vi "VI Tree.vi"   [LabVIEW 2014, in "Agilent NA.lvlib"]
doc: "The VI Tree displays all the user-callable VIs of the instrument driver in an organized table."
uses:
  Agilent NA.lvlib
panel:
  # "NA"
  # "1.0.1"
  # "SEE DIAGRAM\nFOR VI Tree"
  # "© 2014 Agilent Technologies, Inc."
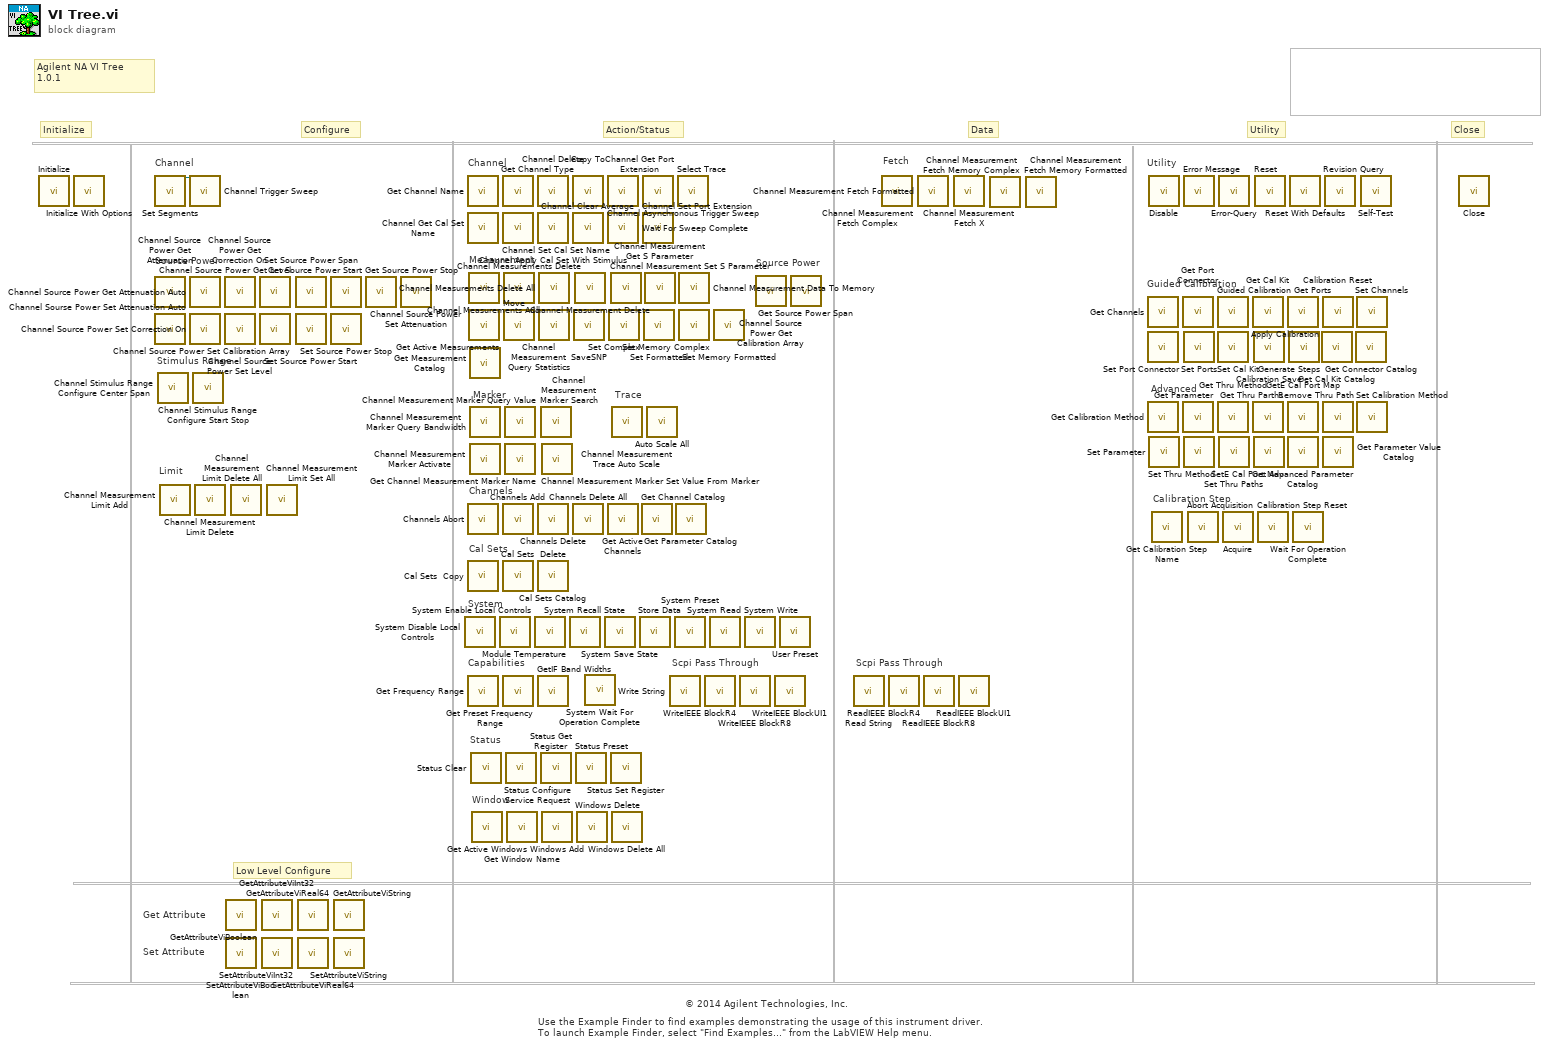
[diagram p0: block diagram]
diagram:
  # "Marker"
  # "Cal Sets"
  # "Utility"
  # "Fetch"
  # "Scpi Pass Through"
  # "Source Power"
  # "Channel"
  # "Status"
  # "Set Attribute"
  # "Get Attribute"
  # "Low Level Configure"
  # "Action/Status"
  # "Agilent NA VI Tree\n1.0.1"
  # "© 2014 Agilent Technologies, Inc."
  # "Close"
  # "Data"
  # "Configure"
  # "Initialize"
  # "Use the Example Finder to find examples demonstrating the usage of this instrument driver.\nTo launch Example Finder, select \"Find Examples...\" from the LabVIEW Help menu."
  # "Window"
  # "Utility"
  # "Scpi Pass Through"
  # "Capabilities"
  # "System"
  # "Calibration Step"
  # "Advanced"
  # "Guided Calibration"
  # "Channels"
  # "Stimulus Range"
  # "Source Power"
  # "Trace"
  # "Limit"
  # "Measurement"
  # "Channel"
  n1 = call "Initialize.vi"() -> ()  [unwired: 10 in, 2 out]
  n2 = call "Initialize With Options.vi"() -> ()  [unwired: 10 in, 2 out]
  n3 = call "Set Segments.vi"() -> ("instrument handle out"=w1:refnum<k15>)  [unwired: 26 in, 1 out]
  n4 = call "Channel Source Power Get Attenuation.vi"() -> ()  [unwired: 9 in, 3 out]
  n5 = call "Channel Sourse Power Set Attenuation Auto.vi"() -> ()  [unwired: 10 in, 2 out]
  n6 = call "Channel Stimulus Range Configure Center Span.vi"() -> ()  [unwired: 10 in, 2 out]
  n7 = call "Channel Measurement Limit Add.vi"() -> ()  [unwired: 10 in, 2 out]
  n8 = call "Channel Trigger Sweep.vi"("instrument handle"=w1) -> ()  [unwired: 9 in, 2 out]
  n9 = call "Channel Source Power Get Attenuation Auto.vi"() -> ()  [unwired: 9 in, 3 out]
  n10 = call "Channel Source Power Set Correction On.vi"() -> ()  [unwired: 10 in, 2 out]
  n11 = call "Channel Stimulus Range Configure Start Stop.vi"() -> ()  [unwired: 10 in, 2 out]
  n12 = call "Channel Measurement Limit Delete.vi"() -> ()  [unwired: 10 in, 2 out]
  n13 = call "Channel Source Power Get Correction On.vi"() -> ()  [unwired: 9 in, 3 out]
  n14 = call "Channel Source Power Set Level.vi"() -> ()  [unwired: 10 in, 2 out]
  n15 = call "GetAttributeViBoolean.vi"() -> ()  [unwired: 9 in, 3 out]
  n16 = call "SetAttributeViBoolean.vi"() -> ()  [unwired: 10 in, 2 out]
  n17 = call "Channel Measurement Limit Delete All.vi"() -> ()  [unwired: 10 in, 2 out]
  n18 = call "Channel Source Power Get Level.vi"() -> ()  [unwired: 9 in, 3 out]
  n19 = call "Channel Source Power Set Calibration Array.vi"() -> ()  [unwired: 9 in, 3 out]
  n20 = call "GetAttributeViInt32.vi"() -> ()  [unwired: 9 in, 3 out]
  n21 = call "SetAttributeViInt32.vi"() -> ()  [unwired: 10 in, 2 out]
  n22 = call "Channel Measurement Limit Set All.vi"() -> ()  [unwired: 26 in, 2 out]
  n23 = call "Set Source Power Span.vi"() -> ()  [unwired: 10 in, 2 out]
  n24 = call "Set Source Power Start.vi"() -> ()  [unwired: 10 in, 2 out]
  n25 = call "GetAttributeViReal64.vi"() -> ()  [unwired: 9 in, 3 out]
  n26 = call "SetAttributeViReal64.vi"() -> ()  [unwired: 10 in, 2 out]
  n27 = call "Get Source Power Start.vi"() -> ()  [unwired: 9 in, 3 out]
  n28 = call "Set Source Power Stop.vi"() -> ()  [unwired: 10 in, 2 out]
  n29 = call "GetAttributeViString.vi"() -> ()  [unwired: 9 in, 3 out]
  n30 = call "SetAttributeViString.vi"() -> ()  [unwired: 10 in, 2 out]
  n31 = call "Get Source Power Stop.vi"() -> ()  [unwired: 9 in, 3 out]
  n32 = call "Channel Source Power Set Attenuation.vi"() -> ()  [unwired: 10 in, 2 out]
  n33 = call "System Disable Local Controls.vi"() -> ()  [unwired: 10 in, 2 out]
  n34 = call "Get Channel Name.vi"() -> ()  [unwired: 9 in, 3 out]
  n35 = call "Channel Get Cal Set Name.vi"() -> ()  [unwired: 9 in, 3 out]
  n36 = call "Channels Abort.vi"() -> ()  [unwired: 10 in, 2 out]
  n37 = call "Cal Sets  Copy.vi"() -> ()  [unwired: 10 in, 2 out]
  n38 = call "Get Frequency Range.vi"() -> ()  [unwired: 8 in, 4 out]
  n39 = call "Channel Measurements Add.vi"() -> ()  [unwired: 9 in, 3 out]
  n40 = call "Get Active Measurements.vi"() -> ()  [unwired: 8 in, 4 out]
  n41 = call "Get Measurement Catalog.vi"() -> ()  [unwired: 9 in, 3 out]
  n42 = call "Channel Measurement Marker Query Bandwidth.vi"() -> ()  [unwired: 6 in, 6 out]
  n43 = call "Channel Measurement Marker Activate.vi"() -> ()  [unwired: 10 in, 2 out]
  n44 = call "Status Clear.vi"() -> ()  [unwired: 10 in, 2 out]
  n45 = call "Get Active Windows.vi"() -> ()  [unwired: 8 in, 4 out]
  n46 = call "System Enable Local Controls.vi"() -> ()  [unwired: 10 in, 2 out]
  n47 = call "Get Channel Type.vi"() -> ()  [unwired: 9 in, 3 out]
  n48 = call "Channel Set Cal Set Name.vi"() -> ()  [unwired: 10 in, 2 out]
  n49 = call "Channels Add.vi"() -> ()  [unwired: 9 in, 3 out]
  n50 = call "Cal Sets  Delete.vi"() -> ()  [unwired: 10 in, 2 out]
  n51 = call "Get Preset Frequency Range.vi"() -> ()  [unwired: 8 in, 4 out]
  n52 = call "Channel Measurements Delete.vi"() -> ()  [unwired: 10 in, 2 out]
  n53 = call "Move.vi"() -> ()  [unwired: 10 in, 2 out]
  n54 = call "Channel Measurement Marker Query Value.vi"() -> ()  [unwired: 8 in, 4 out]
  n55 = call "Get Channel Measurement Marker Name.vi"() -> ()  [unwired: 9 in, 3 out]
  n56 = call "Status Configure Service Request.vi"() -> ()  [unwired: 10 in, 2 out]
  n57 = call "Get Window Name.vi"() -> ()  [unwired: 9 in, 3 out]
  n58 = call "Module Temperature.vi"() -> ()  [unwired: 9 in, 3 out]
  n59 = call "Channel Delete.vi"() -> ()  [unwired: 10 in, 2 out]
  n60 = call "Channel Apply Cal Set With Stimulus.vi"() -> ()  [unwired: 10 in, 2 out]
  n61 = call "Channels Delete.vi"() -> ()  [unwired: 10 in, 2 out]
  n62 = call "Cal Sets Catalog.vi"() -> ()  [unwired: 9 in, 3 out]
  n63 = call "GetIF Band Widths.vi"() -> ()  [unwired: 8 in, 4 out]
  n64 = call "Channel Measurements Delete All.vi"() -> ()  [unwired: 10 in, 2 out]
  n65 = call "Channel Measurement Query Statistics.vi"() -> ()  [unwired: 9 in, 3 out]
  n66 = call "Channel Measurement Marker Search.vi"() -> ()  [unwired: 10 in, 2 out]
  n67 = call "Status Get Register.vi"() -> ()  [unwired: 9 in, 3 out]
  n68 = call "Channel Measurement Marker Set Value From Marker.vi"() -> ()  [unwired: 10 in, 2 out]
  n69 = call "Windows Add.vi"() -> ()  [unwired: 10 in, 2 out]
  n70 = call "System Recall State.vi"() -> ()  [unwired: 10 in, 2 out]
  n71 = call "Copy To.vi"() -> ()  [unwired: 10 in, 2 out]
  n72 = call "Channel Clear Average.vi"() -> ()  [unwired: 10 in, 2 out]
  n73 = call "Channels Delete All.vi"() -> ()  [unwired: 10 in, 2 out]
  n74 = call "SaveSNP.vi"() -> ()  [unwired: 10 in, 2 out]
  n75 = call "Channel Measurement Delete.vi"() -> ()  [unwired: 10 in, 2 out]
  n76 = call "Status Preset.vi"() -> ()  [unwired: 10 in, 2 out]
  n77 = call "Windows Delete.vi"() -> ()  [unwired: 10 in, 2 out]
  n78 = call "System Wait For Operation Complete.vi"() -> ()  [unwired: 10 in, 2 out]
  n79 = call "System Save State.vi"() -> ()  [unwired: 10 in, 2 out]
  n80 = call "Channel Asynchronous Trigger Sweep.vi"() -> ()  [unwired: 10 in, 2 out]
  n81 = call "Wait For Sweep Complete.vi"() -> ()  [unwired: 10 in, 2 out]
  n82 = call "Get Active Channels.vi"() -> ()  [unwired: 8 in, 4 out]
  n83 = call "Set Complex.vi"() -> ()  [unwired: 10 in, 2 out]
  n84 = call "Channel Measurement Set S Parameter.vi"() -> ()  [unwired: 10 in, 2 out]
  n85 = call "Status Set Register.vi"() -> ()  [unwired: 10 in, 2 out]
  n86 = call "Channel Measurement Trace Auto Scale.vi"() -> ()  [unwired: 10 in, 2 out]
  n87 = call "Windows Delete All.vi"() -> ()  [unwired: 10 in, 2 out]
  n88 = call "Store Data.vi"() -> ()  [unwired: 10 in, 2 out]
  n89 = call "Get Channel Catalog.vi"() -> ()  [unwired: 9 in, 3 out]
  n90 = call "Channel Get Port Extension.vi"() -> ()  [unwired: 9 in, 3 out]
  n91 = call "Channel Set Port Extension.vi"() -> ()  [unwired: 10 in, 2 out]
  n92 = call "Set Formatted.vi"() -> ()  [unwired: 10 in, 2 out]
  n93 = call "Channel Measurement Get S Parameter.vi"() -> ()  [unwired: 8 in, 4 out]
  n94 = call "Auto Scale All.vi"() -> ()  [unwired: 10 in, 2 out]
  n95 = call "Write String.vi"() -> ()  [unwired: 10 in, 2 out]
  n96 = call "System Preset.vi"() -> ()  [unwired: 10 in, 2 out]
  n97 = call "Get Parameter Catalog.vi"() -> ()  [unwired: 9 in, 3 out]
  n98 = call "Select Trace.vi"() -> ()  [unwired: 10 in, 2 out]
  n99 = call "Channel Measurement Data To Memory.vi"() -> ()  [unwired: 10 in, 2 out]
  n100 = call "Set Memory Complex.vi"() -> ()  [unwired: 10 in, 2 out]
  n101 = call "WriteIEEE BlockR4.vi"() -> ()  [unwired: 10 in, 2 out]
  n102 = call "System Read.vi"() -> ()  [unwired: 8 in, 4 out]
  n103 = call "Set Memory Formatted.vi"() -> ()  [unwired: 10 in, 2 out]
  n104 = call "WriteIEEE BlockR8.vi"() -> ()  [unwired: 10 in, 2 out]
  n105 = call "System Write.vi"() -> ()  [unwired: 10 in, 2 out]
  n106 = call "Channel Source Power Get Calibration Array.vi"() -> ()  [unwired: 8 in, 4 out]
  n107 = call "WriteIEEE BlockUI1.vi"() -> ()  [unwired: 10 in, 2 out]
  n108 = call "User Preset.vi"() -> ()  [unwired: 10 in, 2 out]
  n109 = call "Get Source Power Span.vi"() -> ()  [unwired: 9 in, 3 out]
  n110 = call "Read String.vi"() -> ()  [unwired: 9 in, 3 out]
  n111 = call "Channel Measurement Fetch Complex.vi"() -> ()  [unwired: 12 in, 4 out]
  n112 = call "ReadIEEE BlockR4.vi"() -> ()  [unwired: 8 in, 4 out]
  n113 = call "Channel Measurement Fetch Formatted.vi"() -> ()  [unwired: 8 in, 4 out]
  n114 = call "ReadIEEE BlockR8.vi"() -> ()  [unwired: 8 in, 4 out]
  n115 = call "Channel Measurement Fetch X.vi"() -> ()  [unwired: 8 in, 4 out]
  n116 = call "ReadIEEE BlockUI1.vi"() -> ()  [unwired: 8 in, 4 out]
  n117 = call "Channel Measurement Fetch Memory Complex.vi"() -> ()  [unwired: 12 in, 4 out]
  n118 = call "Channel Measurement Fetch Memory Formatted.vi"() -> ()  [unwired: 8 in, 4 out]
  n119 = call "Get Channels.vi"() -> ()  [unwired: 8 in, 4 out]
  n120 = call "Set Port Connector.vi"() -> ()  [unwired: 10 in, 2 out]
  n121 = call "Get Calibration Method.vi"() -> ()  [unwired: 9 in, 3 out]
  n122 = call "Disable.vi"() -> ()  [unwired: 10 in, 2 out]
  n123 = call "Set Parameter.vi"() -> ()  [unwired: 10 in, 2 out]
  n124 = call "Get Calibration Step Name.vi"() -> ()  [unwired: 9 in, 3 out]
  n125 = call "Get Port Connector.vi"() -> ()  [unwired: 9 in, 3 out]
  n126 = call "Get Parameter.vi"() -> ()  [unwired: 9 in, 3 out]
  n127 = call "Error Message.vi"() -> ()  [unwired: 9 in, 3 out]
  n128 = call "Set Ports.vi"() -> ()  [unwired: 10 in, 2 out]
  n129 = call "Set Thru Method.vi"() -> ()  [unwired: 10 in, 2 out]
  n130 = call "Abort Acquisition.vi"() -> ()  [unwired: 10 in, 2 out]
  n131 = call "Guided Calibration Get Ports.vi"() -> ()  [unwired: 8 in, 4 out]
  n132 = call "Set Cal Kit.vi"() -> ()  [unwired: 10 in, 2 out]
  n133 = call "Get Thru Method.vi"() -> ()  [unwired: 9 in, 3 out]
  n134 = call "Error-Query.vi"() -> ()  [unwired: 8 in, 4 out]
  n135 = call "Set Thru Paths.vi"() -> ()  [unwired: 10 in, 2 out]
  n136 = call "Acquire.vi"() -> ()  [unwired: 10 in, 2 out]
  n137 = call "Get Cal Kit.vi"() -> ()  [unwired: 9 in, 3 out]
  n138 = call "Get Thru Parths.vi"() -> ()  [unwired: 8 in, 4 out]
  n139 = call "Calibration Save.vi"() -> ()  [unwired: 10 in, 2 out]
  n140 = call "SetE Cal Port Map.vi"() -> ()  [unwired: 10 in, 2 out]
  n141 = call "Reset.vi"() -> ()  [unwired: 10 in, 2 out]
  n142 = call "Calibration Step Reset.vi"() -> ()  [unwired: 10 in, 2 out]
  n143 = call "Apply Calibration.vi"() -> ()  [unwired: 10 in, 2 out]
  n144 = call "GetE Cal Port Map.vi"() -> ()  [unwired: 9 in, 3 out]
  n145 = call "Get Advanced Parameter Catalog.vi"() -> ()  [unwired: 9 in, 3 out]
  n146 = call "Generate Steps.vi"() -> ()  [unwired: 10 in, 2 out]
  n147 = call "Reset With Defaults.vi"() -> ()  [unwired: 10 in, 2 out]
  n148 = call "Wait For Operation Complete.vi"() -> ()  [unwired: 10 in, 2 out]
  n149 = call "Get Cal Kit Catalog.vi"() -> ()  [unwired: 9 in, 3 out]
  n150 = call "Calibration Reset.vi"() -> ()  [unwired: 10 in, 2 out]
  n151 = call "Remove Thru Path.vi"() -> ()  [unwired: 10 in, 2 out]
  n152 = call "Get Parameter Value Catalog.vi"() -> ()  [unwired: 9 in, 3 out]
  n153 = call "Revision Query.vi"() -> ()  [unwired: 8 in, 4 out]
  n154 = call "Get Connector Catalog.vi"() -> ()  [unwired: 9 in, 3 out]
  n155 = call "Set Channels.vi"() -> ()  [unwired: 10 in, 2 out]
  n156 = call "Set Calibration Method.vi"() -> ()  [unwired: 10 in, 2 out]
  n157 = call "Self-Test.vi"() -> ()  [unwired: 8 in, 4 out]
  n158 = call "Close.vi"() -> ()  [unwired: 11 in, 1 out]
